vi "CB Discretize SSM.vi"(11 "Cont SSM":T2) -> (3 "State Space Model":T2)   [LabVIEW 2020]
uses:
  CB State Space.ctl
  <vilib>/Analysis/Matrix/Datatypes/RealMatrix.ctl
  <vilib>/Analysis/Matrix/Numeric/Conversions/Array To Matrix - RA2.vi
  <vilib>/Analysis/Matrix/Numeric/Multiply/Multiply - R,RM.vi
  <vilib>/Analysis/Matrix/Numeric/Exponential/Exponential - RM.vi
  <vilib>/Analysis/Matrix/NI_Matrix.lvlib
panel:
  out "e^A":T1
  out "Bd":T1
  out "Ad":T1
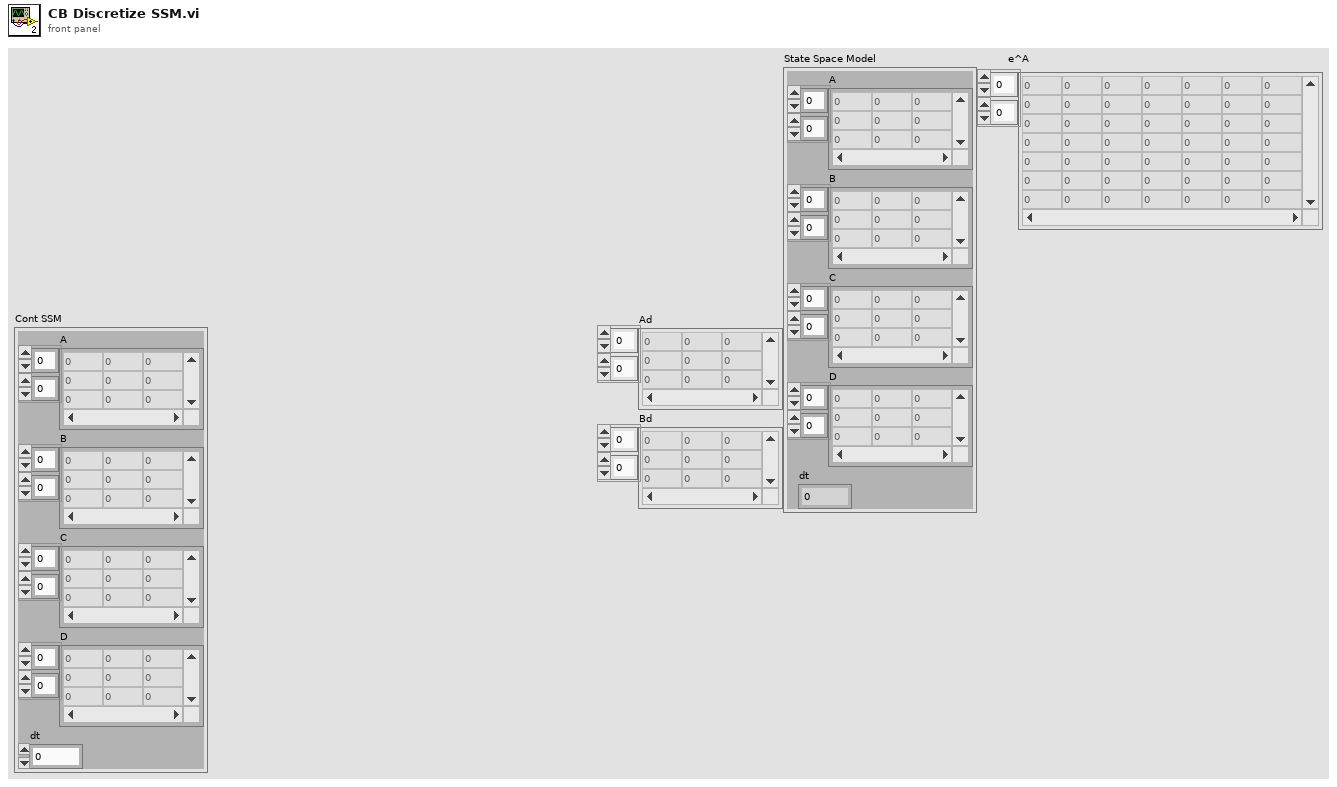
[diagram p1: front panel]
types:
  T1 = typedef "NI_Matrix.lvlib/RealMatrix.ctl" = dbl[][]
  T2 = typedef "CB State Space.ctl" = cluster{"A":T1, "B":T1, "C":T1, "D":T1, "dt":dbl}
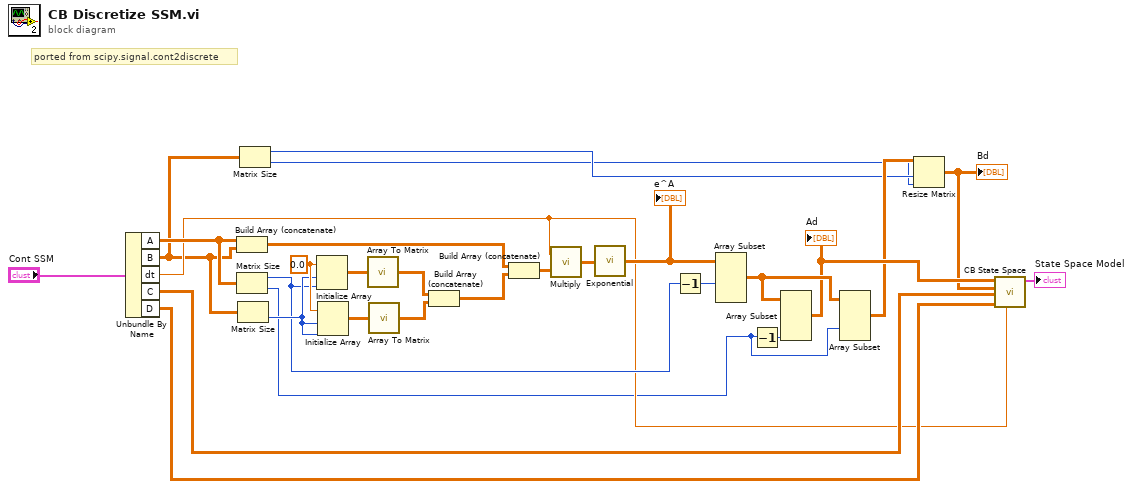
[diagram p0: block diagram]
diagram:
  w26 = 0.0 ("element")
  # "ported from scipy.signal.cont2discrete"
  n1 = Unbundle By Name("Cont SSM") -> ("A"=w27:T1, "B"=w5:T1, "dt"=w9:dbl, "C"=w11:T1, "D"=w10:T1)
  n2 = Build Array (concatenate)(w27, w5) -> (w19:T1)
  n3 = Matrix Size(0:w27) -> (1:w15:i32, 2:w7:i32)
  n4 = Matrix Size(0:w5) -> (2:w25:i32)  [unwired: 1 out]
  n5 = Matrix Size(0:w5) -> (1:w3:i32, 2:w2:i32)
  n6 = Initialize Array(w26, w25, w15) -> (w24:dbl[][])
  n7 = Initialize Array(w26, w25, w25) -> (w23:dbl[][])
  n8 = call-poly <vilib>:"Array To Matrix.vi"("Real 2D Array"=w24) -> ("Real Matrix"=w22:T1)
  n9 = call-poly <vilib>:"Array To Matrix.vi"("Real 2D Array"=w23) -> ("Real Matrix"=w21:T1)
  n10 = Build Array (concatenate)(w22, w21) -> (w20:T1)
  n11 = Build Array (concatenate)(w19, w20) -> (w18:T1)
  n12 = call-poly <vilib>:"Multiply.vi"("Real Matrix A"=w18, "Real Scalar c"=w9) -> ("c * A"=w17:T1)
  n13 = call-poly <vilib>:"Exponential.vi"("Real Matrix A"=w17) -> ("e^A"=w16:T1)
  "e^A" <- w16
  n14 = Decrement(x=w15) -> (x-1=w14:i32)
  n15 = Array Subset(array=w16, length (row)=w14) -> (w13:T1)  [unwired: 3 in]
  n16 = Decrement(x=w7) -> (x-1=w6:i32)
  n17 = Array Subset(array=w13, length (col)=w6) -> (w12:T1)  [unwired: 3 in]
  "Ad" <- w12
  n18 = Array Subset(array=w13, index (col)=w7) -> (w4:T1)  [unwired: 3 in]
  n19 = Resize Matrix(1:w2, 2:w3, 4:w4) -> (0:w1:T1)
  "Bd" <- w1
  n20 = call "CB State Space.vi"("dt"=w9, "D"=w10, "C"=w11, "B"=w1, "A"=w12) -> ("State Space Model"=→"State Space Model":T2)  [unwired: 5 in, 1 out]
